vi "TTA_MATLAB_Get_Selected_RFICs.vi"(11 "error in":errorcluster) -> (4 "RFICs":i32[](array[numeric]), 15 "error out":errorcluster)   [LabVIEW 2016]
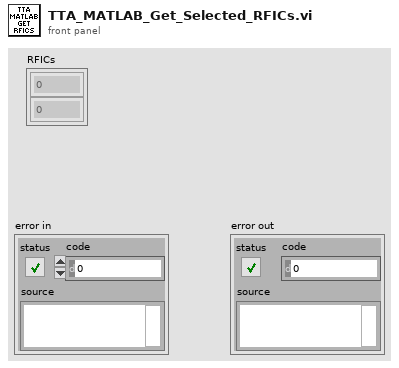
[diagram p1: front panel]
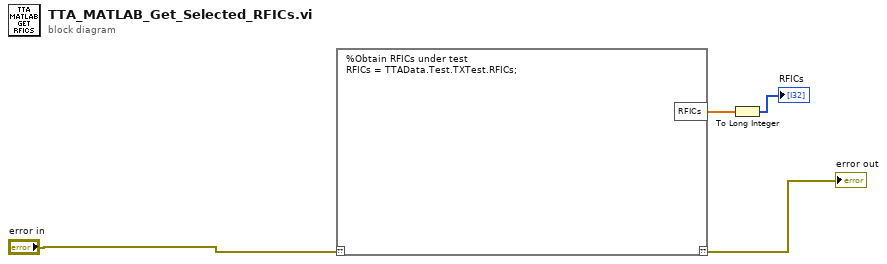
[diagram p0: block diagram]
diagram:
  n1 = script code="%Obtain RFICs under test\nRFICs = TTAData.Test.TXTest.RFICs;"("??"="error in") -> ("??"=→"error out":errorcluster, "RFICs"=w4:dbl[])
  n2 = To Long Integer(number=w4) -> (32bit integer=→"RFICs":i32[])
